vi "Do.vi"(8 "error in":errorcluster, 10 "Input":variant, 11 "ITask Actor in":refnum<class "ITask Actor.lvclass">) -> (0 "error out":errorcluster, 3 "ITask Actor out":refnum<class "ITask Actor.lvclass">)   [LabVIEW 2023, in "ITask Actor.lvlib" / "ITask Actor.lvclass"]
uses:
  ITask Actor.lvclass
  <vilib>/Utility/error.llb/Error Cluster From Error Code.vi
  <vilib>/ErrorRing/Error Ring.xnode
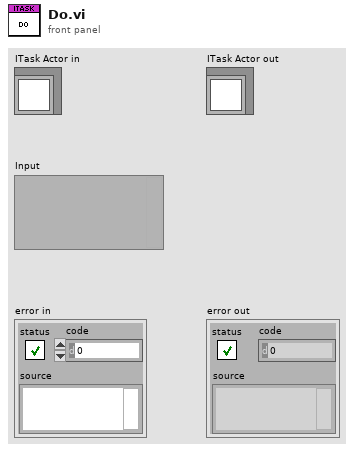
[diagram p1: front panel]
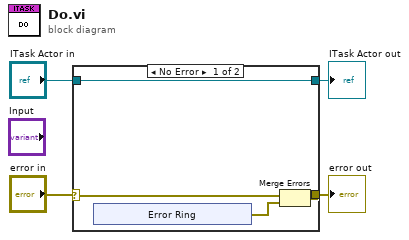
[diagram p0: block diagram]
diagram:
  n1 = case shown="No Error" "error in" {
    selector: "error in" -> [w6 w15]
    tunnel: [w8 w15] -> w4
    tunnel: "ITask Actor in" -> [w5 w14]
    tunnel: [w5 w14] -> w1
    frame No Error {
      n2 = xnode "Error Ring"() -> ("error out"=w7:errorcluster)
      n3 = Merge Errors(w6, w7) -> (w8:errorcluster)
    }
    frame Error {
    }
  }
  "error out" <- w4
  "ITask Actor out" <- w1
